vi "demandsView.vi"(10 "UserEvents in":refnum<class "UserEvents.lvclass">) -> ()   [LabVIEW 2013, in "FAMTViews.lvlib"]
uses:
  FAMTViews.lvlib
  UserEvents/UserEvents.lvclass
  Typedefs/ForceSetpoint.ctl
  CommandFactory/CommandFactory.lvclass
  UserEvents/UserEvents.lvclass/UserEvents.ctl
  Typedefs/StateSelector.ctl
  Typedefs/CommandSelector.ctl
  Commands/ForceSetpoint/ForceSetpoint.lvclass
  Commands/ForceSetpoint/ForceSetpoint.lvclass/ForceSetpoint.ctl
  Typedefs/FAMTTypedefs.lvlib
  ConfigurationTestParameters/ConfigurationTestParameters.lvclass
panel:
  in  "enableMotionIsTrue":bool
  in  "sendForceDemandIsTrue":bool
  in  "stopMotionIsTrue":bool
  in  "stopAutomatedTestIsTrue":bool
  in  "startAutomatedTestIsTrue":bool
  in  "Force Demand":T1 min=-888.0 max=888.0 format="%.2f"
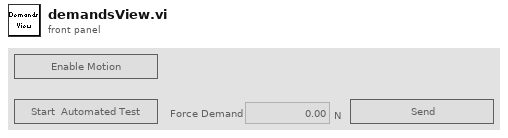
[diagram p1: front panel]
types:
  T1 = typedef "FAMTTypedefs.lvlib/ForceSetpoint.ctl" = dbl[unit]
  T2 = enum8{"Enabled", "Disabled", "Disabled and Grayed Out"}
  T3 = typedef "FAMTTypedefs.lvlib/PubDataEvents.ctl" = cluster{"State":refnum<user-event>, "ErrorCode":refnum<user-event>, "OutputData":refnum<user-event>, "InputData":refnum<user-event>, "ControllerData":refnum<user-event>, "TestStatus":refnum<user-event>, "LogPath":refnum<user-event>}
  T4 = typedef "FAMTTypedefs.lvlib/SubDataEvents.ctl" = cluster{"Command":refnum<user-event>}
  T5 = cluster{"Event Registration Refnum":refnum<event-registration>}
  T6 = typedef "FAMTTypedefs.lvlib/StateSelector.ctl" = enum16{"EndingCycleState", "FaultState", "InteractiveSetpointState", "OffState", "StandbyState", "StoppedState"}
  T7 = typedef "FAMTTypedefs.lvlib/CommandSelector.ctl" = enum16{"ClearError", "EnableCompensator", "Exit", "ForceSetpoint", "StandBy", "Start", "StartAutomatedTest", "StopAutomatedTest", "StopCompensator", "Update"}
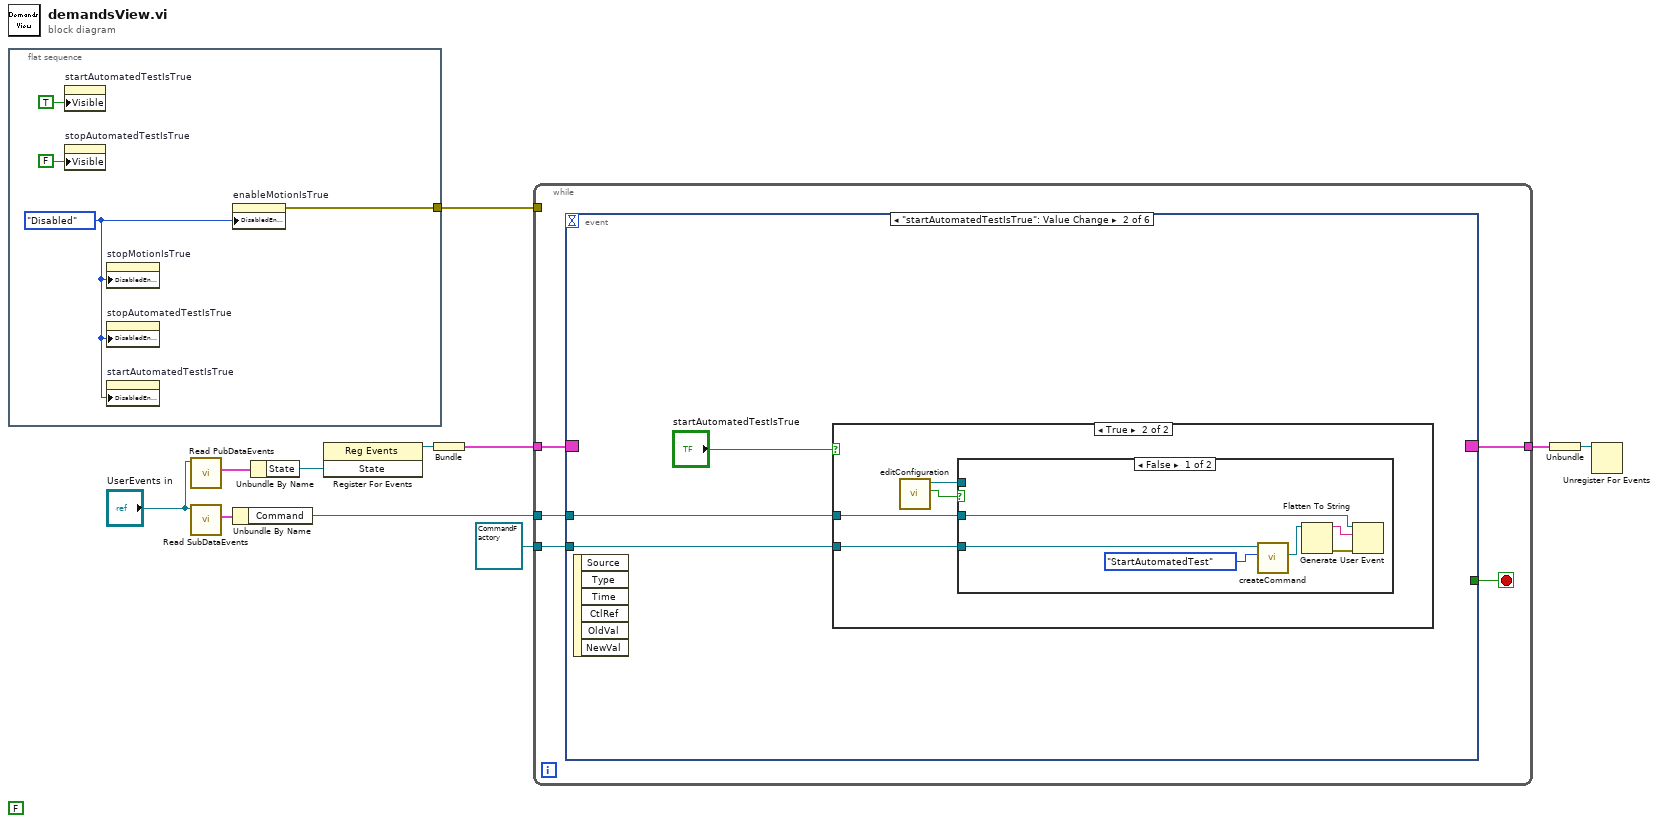
[diagram p0: block diagram]
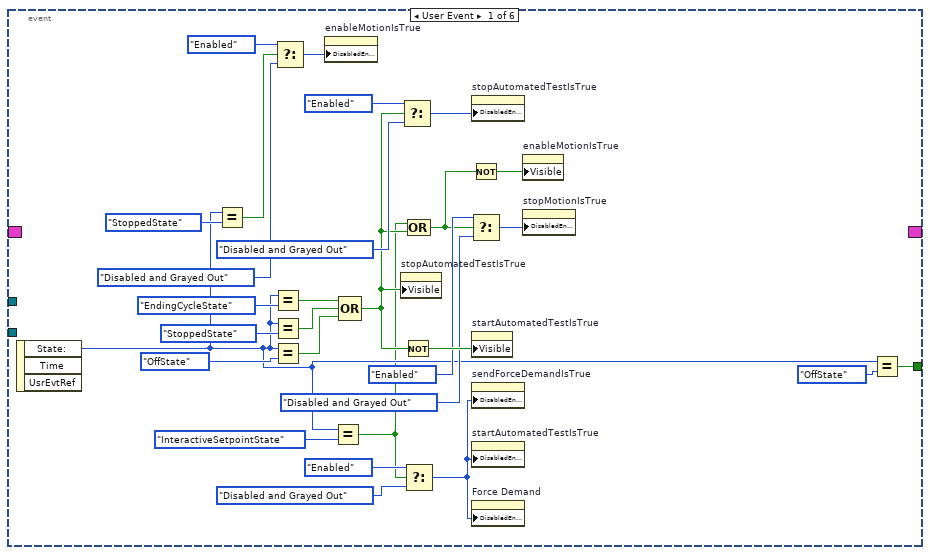
[diagram p2: hidden frame]
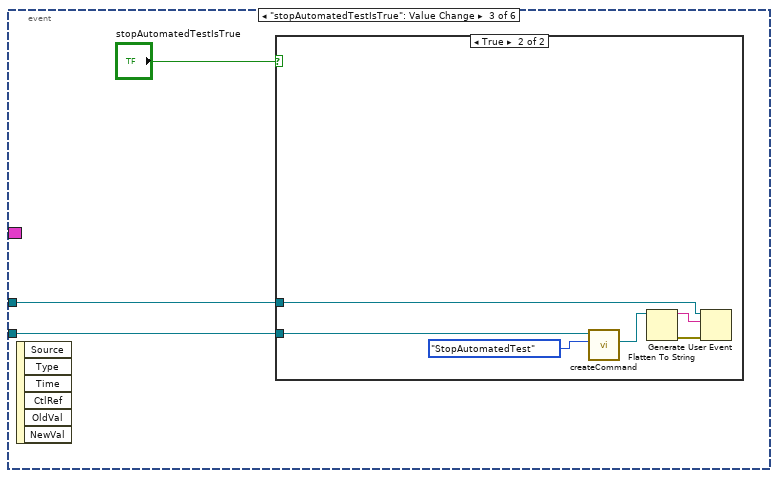
[diagram p5: hidden frame]
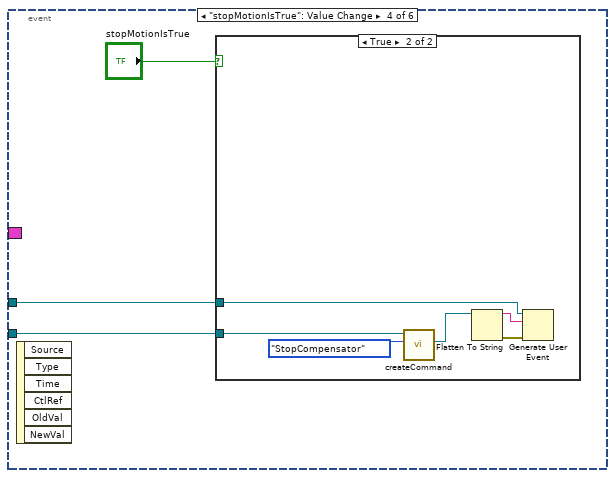
[diagram p7: hidden frame]
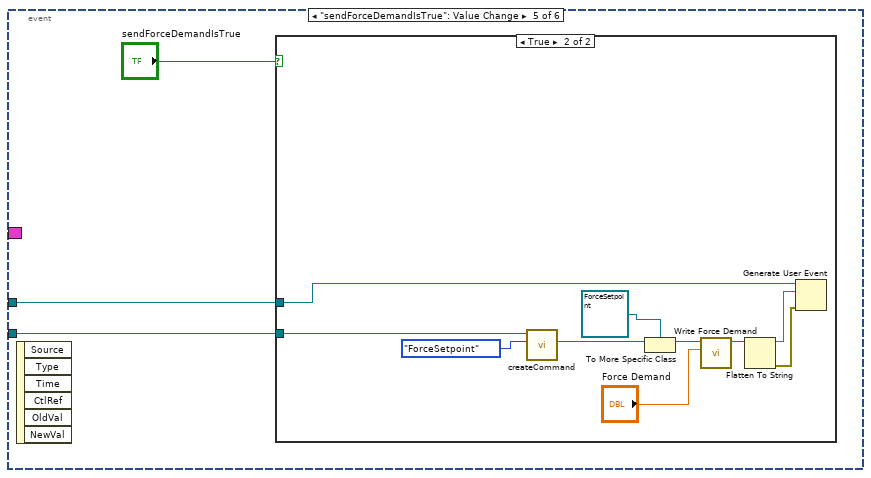
[diagram p9: hidden frame]
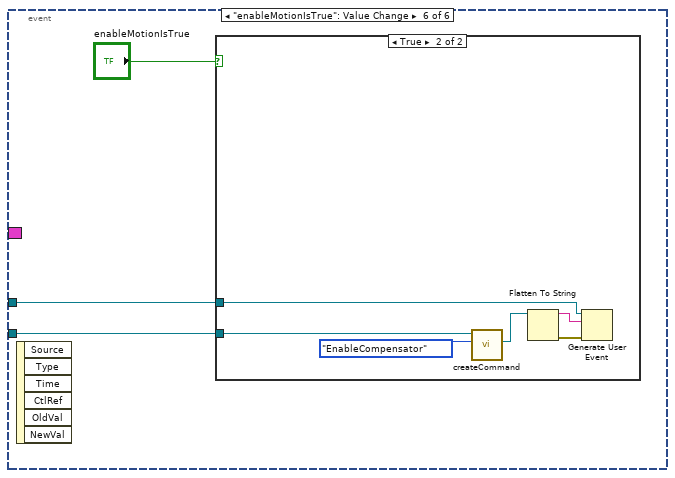
[diagram p11: hidden frame]
diagram:
  (unwired) FALSE ("motionInProgress")
  n1 = flat-sequence {
    tunnel: [w12] -> w1
    frame #0 {
      w15 = T2."Disabled" ("Disabled")
      n2 = property on="startAutomatedTestIsTrue" class="Bool"("Visible"=TRUE) -> ()  [unwired: 2 in, 2 out]
      n3 = property on="stopAutomatedTestIsTrue" class="Bool"("Visible"=FALSE) -> ()  [unwired: 2 in, 2 out]
      n4 = property on="stopMotionIsTrue" class="Bool"("DisabledEnum"=w15) -> ()  [unwired: 2 in, 2 out]
      n5 = property on="stopAutomatedTestIsTrue" class="Bool"("DisabledEnum"=w15) -> ()  [unwired: 2 in, 2 out]
      n6 = property on="startAutomatedTestIsTrue" class="Bool"("DisabledEnum"=w15) -> ()  [unwired: 2 in, 2 out]
      n7 = property on="enableMotionIsTrue" class="Bool"("DisabledEnum"=w15) -> (error out=w12:errorcluster)  [unwired: 2 in, 1 out]
    }
  }
  n8 = call "Read PubDataEvents.vi"("UserEvents in"="UserEvents in") -> ("PubDataEvents"=w8:T3)  [unwired: 9 in, 1 out]
  n9 = call "Read SubDataEvents.vi"("UserEvents in"="UserEvents in") -> ("SubDataEvents"=w9:T4)  [unwired: 9 in, 1 out]
  n10 = Unbundle By Name(w9) -> ("Command"=w6:refnum<user-event>)
  n11 = Unbundle By Name(w8) -> ("State"=w10:refnum<user-event>)
  n12 = register-events(w10) -> (reference out=w11:refnum<event-registration>)  [unwired: 2 in, 1 out]
  n13 = Bundle("Event Registration Refnum"=w11) -> (w7:T5)  [unwired: 1 in]
  n14 = while {
    tunnel: w7 -> [w20]
    tunnel: w6 -> [w19]
    tunnel: [w18] -> w5
    tunnel: refnum<class "CommandFactory.lvclass"> refnum ("CommandFactory.lvclass") -> [w16]
    tunnel: w1 -> [_]
    stop <- w17 stop-if-true
    n15 = event shown="[1] \"startAutomatedTestIsTrue\": Value Change" {
      selector: w20 -> [_ _ _ _ _ _]
      dyn-events: [_ _ _ _ _ _] -> w18
      timeout: _ -> [_ _ _ _ _ _]
      tunnel: w19 -> [_ w50 w65 w73 w83 w96]
      tunnel: [w46 _ _ _ _ _] -> w17
      tunnel: w16 -> [_ w51 w64 w72 w82 w95]
      event User Event {
        n16 = event-data() -> ("State:"=w26:T6)  [unwired: 1 in, 2 out]
        n17 = Equal?(x=w26, y=StateSelector."StoppedState") -> (x = y?=w23:bool)
        n18 = Equal?(x=w26, y=StateSelector."EndingCycleState") -> (x = y?=w37:bool)
        n19 = Equal?(x=w26, y=StateSelector."StoppedState") -> (x = y?=w36:bool)
        n20 = Equal?(x=w26, y=StateSelector."OffState") -> (x = y?=w35:bool)
        n21 = Select(t=T2."Enabled" ("Disabled"), s=w23, f=T2."Disabled and Grayed Out" ("Disabled")) -> (s? t:f=w45:T2)
        n22 = property on="enableMotionIsTrue" class="Bool"("DisabledEnum"=w45) -> ()  [unwired: 2 in, 2 out]
        n23 = Equal?(x=w26, y=StateSelector."InteractiveSetpointState") -> (x = y?=w25:bool)
        n24 = Compound Arithmetic op=OR(w37, w36, w35) -> (w30:bool)
        n25 = property on="stopAutomatedTestIsTrue" class="Bool"("Visible"=w30) -> ()  [unwired: 2 in, 2 out]
        n26 = Select(t=T2."Enabled" ("Disabled"), s=w30, f=T2."Disabled and Grayed Out" ("Disabled")) -> (s? t:f=w33:T2)
        n27 = Not(x=w30) -> (.not. x?=w31:bool)
        n28 = Select(t=T2."Enabled" ("Disabled"), s=w25, f=T2."Disabled and Grayed Out" ("Disabled")) -> (s? t:f=w24:T2)
        n29 = Compound Arithmetic op=OR(w25, w30) -> (w21:bool)
        n30 = Not(x=w21) -> (.not. x?=w22:bool)
        n31 = Select(t=T2."Enabled" ("Disabled"), s=w21, f=T2."Disabled and Grayed Out" ("Disabled")) -> (s? t:f=w28:T2)
        n32 = property on="stopAutomatedTestIsTrue" class="Bool"("DisabledEnum"=w33) -> ()  [unwired: 2 in, 2 out]
        n33 = property on="startAutomatedTestIsTrue" class="Bool"("Visible"=w31) -> ()  [unwired: 2 in, 2 out]
        n34 = property on="sendForceDemandIsTrue" class="Bool"("DisabledEnum"=w24) -> ()  [unwired: 2 in, 2 out]
        n35 = property on="startAutomatedTestIsTrue" class="Bool"("DisabledEnum"=w24) -> ()  [unwired: 2 in, 2 out]
        n36 = property on="Force Demand" class="DigNum (strict)"("DisabledEnum"=w24) -> ()  [unwired: 2 in, 2 out]
        n37 = property on="enableMotionIsTrue" class="Bool"("Visible"=w22) -> ()  [unwired: 2 in, 2 out]
        n38 = property on="stopMotionIsTrue" class="Bool"("DisabledEnum"=w28) -> ()  [unwired: 2 in, 2 out]
        n39 = Equal?(x=w26, y=StateSelector."OffState") -> (x = y?=w46:bool)
      }
      event "startAutomatedTestIsTrue": Value Change {
        n40 = event-data() -> ()  [unwired: 1 in, 6 out]
        n41 = case shown="True" "startAutomatedTestIsTrue" {
          tunnel: w51 -> [_ w56]
          tunnel: w50 -> [_ w55]
          frame False {
          }
          frame True {
            n42 = call "editConfiguration.vi"() -> ("cancelIsTrue out"=w53:bool, "ConfigurationThisComponent out"=w54:refnum<class "ConfigurationTestParameters.lvclass">)  [unwired: 9 in, 1 out]
            n43 = case shown="False" w53 {
              tunnel: w56 -> [w62 _]
              tunnel: w55 -> [w58 _]
              tunnel: w54 -> [_ _]
              frame False {
                n44 = call-dynamic "createCommand.vi"("Command"=CommandSelector."StartAutomatedTest", "CommandFactory in"=w62) -> ("command"=w57:refnum<class "Command.lvclass">)  [unwired: 7 in, 2 out]
                n45 = Flatten To String(anything=w57) -> (data string=w59:string, error out=w60:errorcluster)  [unwired: 3 in, 1 out]
                n46 = Generate User Event(user event=w58, event data cluster=w59, error in=w60) -> ()  [unwired: 1 in, 2 out]
              }
              frame True {
              }
            }
          }
        }
      }
      event "stopAutomatedTestIsTrue": Value Change {
        n47 = event-data() -> ()  [unwired: 1 in, 6 out]
        n48 = case shown="True" "stopAutomatedTestIsTrue" {
          tunnel: w64 -> [_ w71]
          tunnel: w65 -> [_ w67]
          frame False {
          }
          frame True {
            n49 = call-dynamic "createCommand.vi"("Command"=CommandSelector."StopAutomatedTest", "CommandFactory in"=w71) -> ("command"=w66:refnum<class "Command.lvclass">)  [unwired: 7 in, 2 out]
            n50 = Flatten To String(anything=w66) -> (data string=w68:string, error out=w69:errorcluster)  [unwired: 3 in, 1 out]
            n51 = Generate User Event(user event=w67, event data cluster=w68, error in=w69) -> ()  [unwired: 1 in, 2 out]
          }
        }
      }
      event "stopMotionIsTrue": Value Change {
        n52 = event-data() -> ()  [unwired: 1 in, 6 out]
        n53 = case shown="True" "stopMotionIsTrue" {
          tunnel: w72 -> [_ w80]
          tunnel: w73 -> [_ w76]
          frame False {
          }
          frame True {
            n54 = call-dynamic "createCommand.vi"("Command"=CommandSelector."StopCompensator", "CommandFactory in"=w80) -> ("command"=w75:refnum<class "Command.lvclass">)  [unwired: 7 in, 2 out]
            n55 = Flatten To String(anything=w75) -> (data string=w77:string, error out=w78:errorcluster)  [unwired: 3 in, 1 out]
            n56 = Generate User Event(user event=w76, event data cluster=w77, error in=w78) -> ()  [unwired: 1 in, 2 out]
          }
        }
      }
      event "sendForceDemandIsTrue": Value Change {
        n57 = event-data() -> ()  [unwired: 1 in, 6 out]
        n58 = case shown="True" "sendForceDemandIsTrue" {
          tunnel: w82 -> [_ w93]
          tunnel: w83 -> [_ w89]
          frame False {
          }
          frame True {
            n59 = call-dynamic "createCommand.vi"("Command"=CommandSelector."ForceSetpoint", "CommandFactory in"=w93) -> ("command"=w88:refnum<class "Command.lvclass">)  [unwired: 7 in, 2 out]
            n60 = To More Specific Class(target class=refnum<class "ForceSetpoint.lvclass"> refnum ("ForceDemand.lvclass"), reference=w88) -> (specific class reference=w86:refnum<class "ForceSetpoint.lvclass">)  [unwired: 1 in, 1 out]
            n61 = call "Write Force Demand.vi"("Force Setpoint"="Force Demand", "ForceSetpoint in"=w86) -> ("ForceSetpoint out"=w85:refnum<class "ForceSetpoint.lvclass">)  [unwired: 9 in]
            n62 = Flatten To String(anything=w85) -> (data string=w90:string, error out=w91:errorcluster)  [unwired: 3 in, 1 out]
            n63 = Generate User Event(user event=w89, event data cluster=w90, error in=w91) -> ()  [unwired: 1 in, 2 out]
          }
        }
      }
      event "enableMotionIsTrue": Value Change {
        n64 = event-data() -> ()  [unwired: 1 in, 6 out]
        n65 = case shown="True" "enableMotionIsTrue" {
          tunnel: w95 -> [_ w102]
          tunnel: w96 -> [_ w98]
          frame False {
          }
          frame True {
            n66 = call-dynamic "createCommand.vi"("Command"=CommandSelector."EnableCompensator", "CommandFactory in"=w102) -> ("command"=w97:refnum<class "Command.lvclass">)  [unwired: 7 in, 2 out]
            n67 = Flatten To String(anything=w97) -> (data string=w99:string, error out=w100:errorcluster)  [unwired: 3 in, 1 out]
            n68 = Generate User Event(user event=w98, event data cluster=w99, error in=w100) -> ()  [unwired: 1 in, 2 out]
          }
        }
      }
    }
  }
  n69 = Unbundle(w5) -> ("Event Registration Refnum"=w4:refnum<event-registration>)
  n70 = Unregister For Events(event registration refnum=w4) -> ()  [unwired: 1 in, 1 out]
